vi "initialize.vi"(8 "error in (no error)":errorcluster, 11 "CM_State Machine in":refnum<class "CM_State Machine.lvclass">) -> (0 "error out":errorcluster, 3 "CM_State Machine out":refnum<class "CM_State Machine.lvclass">)   [LabVIEW 2018, in "CM_State Machine.lvclass"]
uses:
  CM_State Machine.lvclass
  CM_State Machine.lvclass/CM_State Machine.ctl
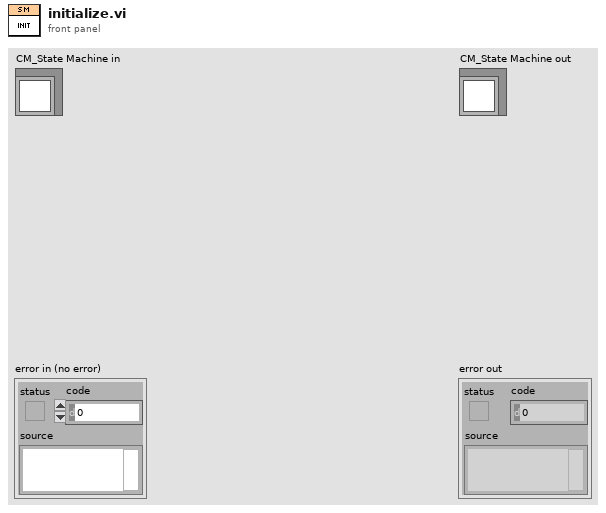
[diagram p1: front panel]
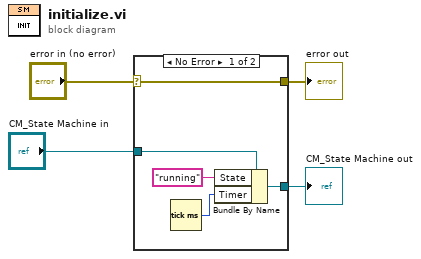
[diagram p0: block diagram]
diagram:
  n1 = case shown="No Error" "error in (no error)" {
    selector: "error in (no error)" -> [w9 w11]
    tunnel: [w9 w11] -> w3
    tunnel: [w5 w10] -> w1
    tunnel: "CM_State Machine in" -> [w8 w10]
    frame No Error {
      n2 = Tick Count (ms)() -> (millisecond timer value=w6:u32)
      n3 = Bundle By Name(cluster=w8, "State"="running", "Timer"=w6) -> (w5:refnum<class "CM_State Machine.lvclass">)
    }
    frame Error {
    }
  }
  "error out" <- w3
  "CM_State Machine out" <- w1
